vi "CalcSample.vi"(8 "error in (no error)":errorcluster, 11 "MultiBandState in":refnum<class "MultiBandState.lvclass">) -> (0 "error out":errorcluster, 3 "MultiBandState out":refnum<class "MultiBandState.lvclass">)   [LabVIEW 2014, in "Functions.lvlib" / "MultiBandState.lvclass"]
uses:
  MultiBandState.lvclass
  MultiBandState.lvclass/MultiBandState.ctl
  FunctionBaseClass/FunctionBase.lvclass/FunctionBase.ctl
  <vilib>/Analysis/baseanly.llb/Real A x B.vi
  Accessors/Read MultiBand.vi
  FunctionBaseClass/Accessors/Read Waveforms.vi
  Accessors/Write MultiBand.vi
  FunctionBaseClass/Accessors/Write Waveforms.vi
  <vilib>/Analysis/NI_AALBase.lvlib
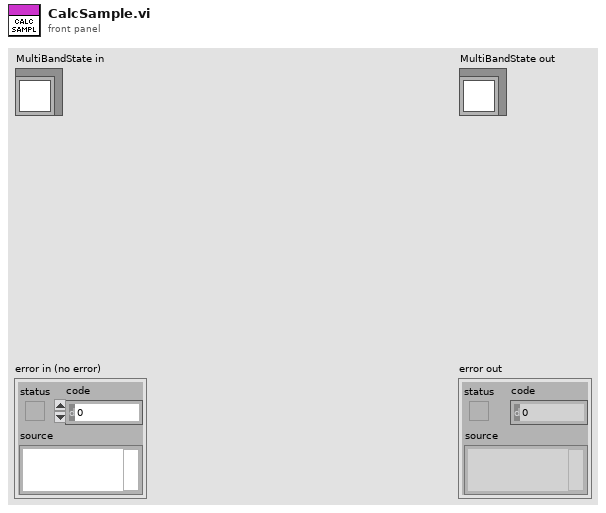
[diagram p1: front panel]
types:
  T1 = typedef "NI_Matrix.lvlib/RealMatrix.ctl" = dbl[][]
  T2 = cluster{"Handle":string, "Size":i32, "Gain":dbl, "Offset":dbl, "A":T1, "B":T1, "C":T1, "D":T1, "X":T1, "Waveform":waveform(dbl)}[]
  T3 = cluster{"Handle":string, "Size":i32, "Gain":dbl, "Offset":dbl, "A":T1, "B":T1, "C":T1, "D":T1, "X":T1, "Waveform":waveform(dbl)}
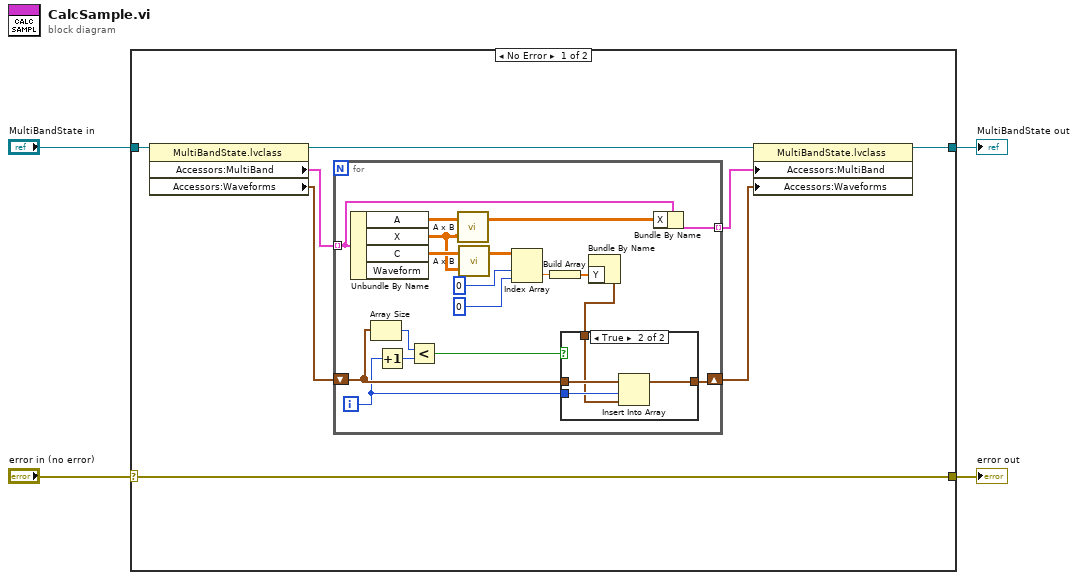
[diagram p0: block diagram]
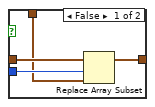
[diagram p2: hidden frame]
diagram:
  n1 = case shown="No Error" "error in (no error)" {
    selector: "error in (no error)" -> [w7 w40]
    tunnel: [w7 w40] -> w3
    tunnel: [w9 w39] -> w1
    tunnel: "MultiBandState in" -> [w12 w39]
    frame No Error {
      n2 = property class="MultiBandState.lvclass"(reference=w12) -> (reference out=w11:refnum<class "MultiBandState.lvclass">, "Accessors:MultiBand"=w10:T2, "Accessors:Waveforms"=w6:waveform(dbl)[])  [unwired: 1 in, 1 out]
      n3 = for {
        tunnel: w10 -> [w30] mode=indexing
        tunnel: [w28] -> w8 mode=indexing
        shift-right: [w13] -> w5
        shift-left: w6 -> [w19]
        i -> [w18]
        n4 = Unbundle By Name(w30) -> ("A"=w21:T1, "X"=w20:T1, "C"=w22:T1)  [unwired: 1 out]
        n5 = Array Size(array=w19) -> (size(s)=w16:i32)
        n6 = Increment(x=w18) -> (x+1=w17:i32)
        n7 = Less?(x=w16, y=w17) -> (x < y?=w15:bool)
        n8 = call-poly <vilib>:"A x B.vi"("B"=w20, "A"=w21) -> ("A x B"=w29:T1)  [unwired: 1 out]
        n9 = call-poly <vilib>:"A x B.vi"("B"=w20, "A"=w22) -> ("A x B"=w27:T1)  [unwired: 1 out]
        n10 = Index Array(array=w27, index (row)=0, index (col)=0 ("index (row)")) -> (element=w24:dbl)
        n11 = Build Array(w24) -> (w23:dbl[])
        n12 = Bundle By Name("Y"=w23) -> (w14:waveform(dbl))  [unwired: 1 in]
        n13 = case shown="True" w15 {
          tunnel: w19 -> [w34 w37]
          tunnel: w18 -> [w33 w38]
          tunnel: w14 -> [w32 w36]
          tunnel: [w31 w35] -> w13
          frame False {
            n14 = Replace Array Subset(array=w34, new element=w32, index=w33) -> (w31:waveform(dbl)[])
          }
          frame True {
            n15 = Insert Into Array(array=w37, index=w38, new element=w36) -> (w35:waveform(dbl)[])
          }
        }
        n16 = Bundle By Name(cluster=w30, "X"=w29) -> (w28:T3)
      }
      n17 = property class="MultiBandState.lvclass"(reference=w11, "Accessors:MultiBand"=w8, "Accessors:Waveforms"=w5) -> (reference out=w9:refnum<class "MultiBandState.lvclass">)  [unwired: 1 in, 1 out]
    }
    frame Error {
    }
  }
  "error out" <- w3
  "MultiBandState out" <- w1
